vi "Generate Power Spac from RAW-Stream.vi"() -> ()   [LabVIEW 2016]
uses:
  <vilib>/measure/maspectr.llb/FFT Power Spectrum and PSD for 1 Chan (CDB).vi
  <vilib>/measure/NI_MAPro.lvlib
panel:
  out "Power Spectrum":cluster{"f0":dbl, "df":dbl, "magnitude":dbl[]}[](graph)
  in  "Channel File 3":cluster{"File Path":path, "Simulate Data":bool}
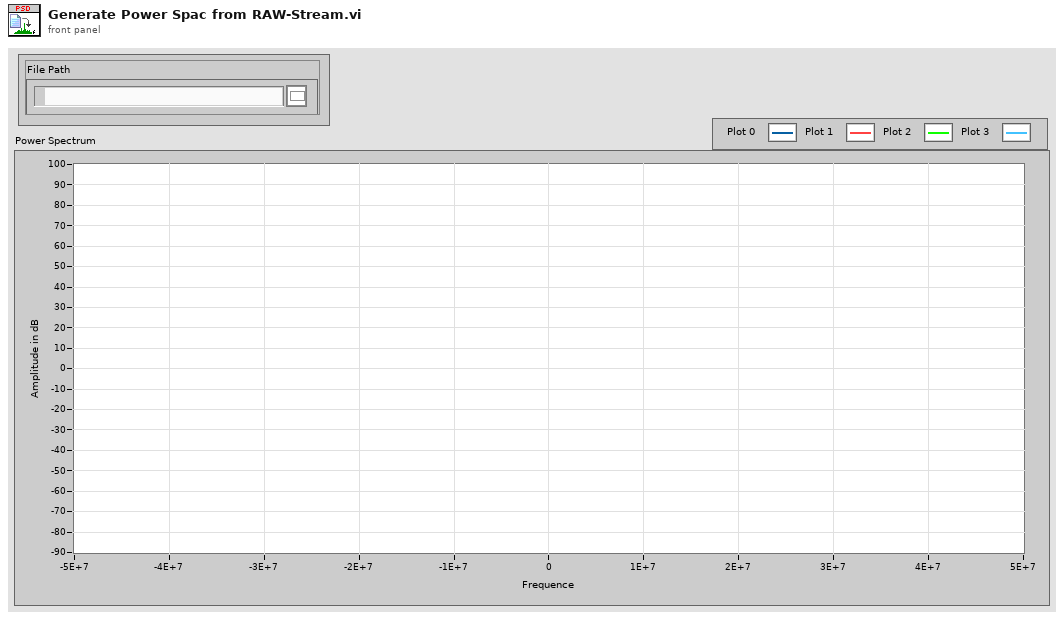
[diagram p1: front panel]
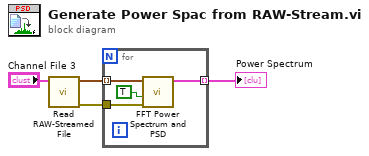
[diagram p0: block diagram]
diagram:
  n1 = call "Read RAW-Streamed File.vi"("Channel File 3"="Channel File 3") -> ("error out"=w2:errorcluster, "Array"=w3:waveform(cdb)[])  [unwired: 9 in]
  n2 = for {
    tunnel: w3 -> [w7] mode=indexing
    tunnel: [w8] -> w1 mode=indexing
    tunnel: w2 -> [w5]
    n3 = call-poly <vilib>:"FFT Power Spectrum and PSD.vi"("error in (no error)"=w5, "dB On (F)"=TRUE ("dB On (T)"), "time signal"=w7) -> ("Power Spectrum / PSD"=w8:cluster{"f0":dbl, "df":dbl, "magnitude":dbl[]})  [unwired: 5 in, 3 out]
  }
  "Power Spectrum" <- w1
